vi "Resolution.vi"(7 "Function":i32(ring), 8 "error in (no error)":errorcluster, 10 "Resolution":u16, 11 "Digtal Multimeter in":refnum<class "Agilent 344xxA.lvclass">) -> (0 "error out":errorcluster, 3 "Digtal Multimeter out":refnum<class "Agilent 344xxA.lvclass">)   [LabVIEW 2020, in "Agilent 344xxA.lvclass"]
uses:
  Agilent 344xxA.lvclass
  Digital Multimeter.lvclass
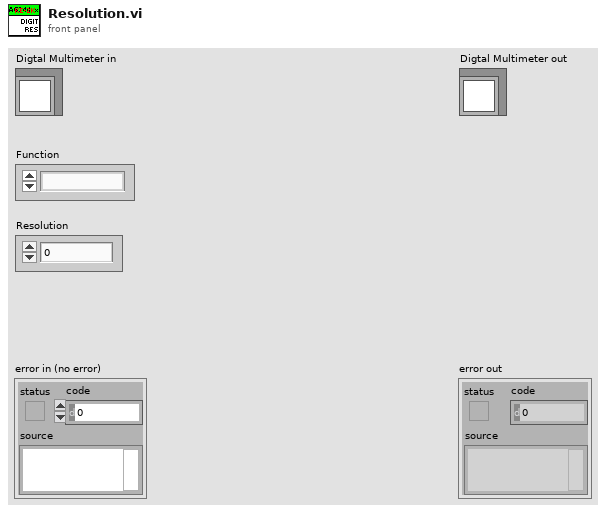
[diagram p1: front panel]
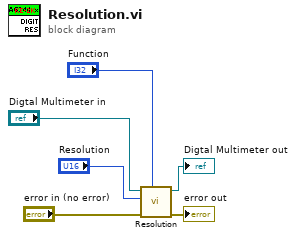
[diagram p0: block diagram]
diagram:
  n1 = call-parent "Resolution.vi"("Function"="Function", "error in (no error)"="error in (no error)", "Resolution"="Resolution", "Digtal Multimeter in"="Digtal Multimeter in") -> ("error out"=→"error out":errorcluster, "Digtal Multimeter out"=→"Digtal Multimeter out":refnum<class "Agilent 344xxA.lvclass">)  [unwired: 6 in]
